vi "Setting GUI.vi"(3 "Path_In":path=path "C:/Users/mclmcgill/Desktop/Stroke_Perceptual_Testing") -> (0 "error out":errorcluster)   [LabVIEW 2012]
uses:
  Global_var.vi
  <userlib>/dhd_sdk7/dhd_sdk7.lvlib
panel:
  in  "Extreme Direction":u8=45 max=40 step=5
  in  "Get_center":bool
  out "Message":string
  out "after_str":string
  out "cur_path":path
  out "Center":dbl[](array[numeric]) format="%#_3g"
  in  "Alignment":bool
  in  "Quit":bool
  in  "Load":bool
  in  "Save":bool
  in  "Language":bool
  in  "Movement Distance":u8=15 max=40 step=5
  in  "Participant's Last Name":string
  in  "Participant's First Name":string
  # "cm"
  # "Recorded Center Position"
  # "degree"
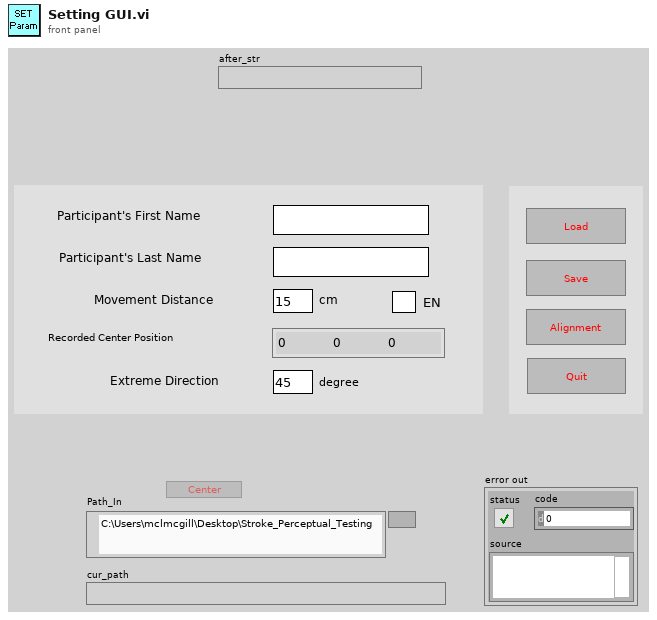
[diagram p1: front panel]
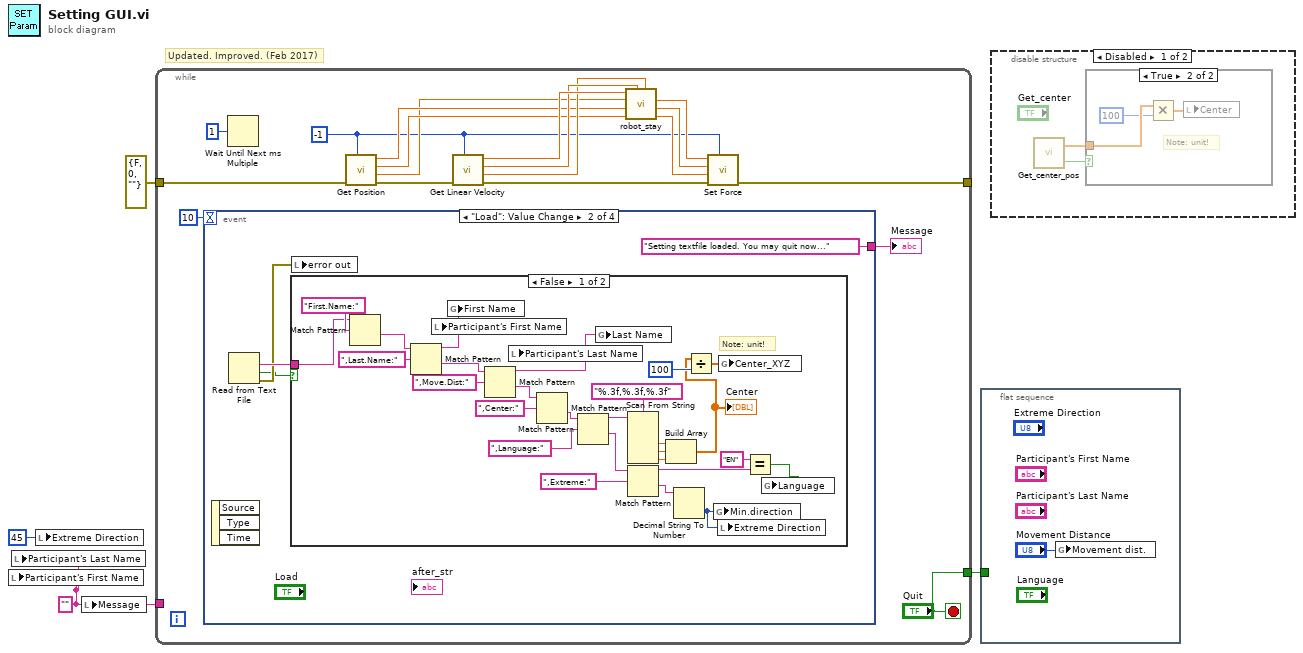
[diagram p0: block diagram]
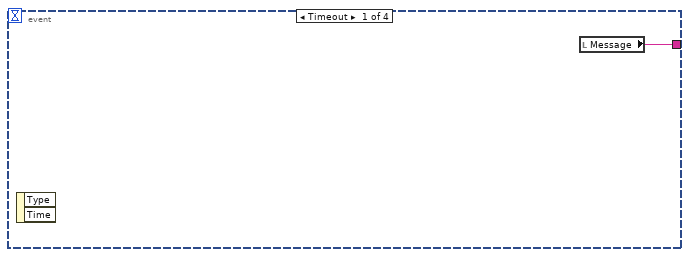
[diagram p4: hidden frame]
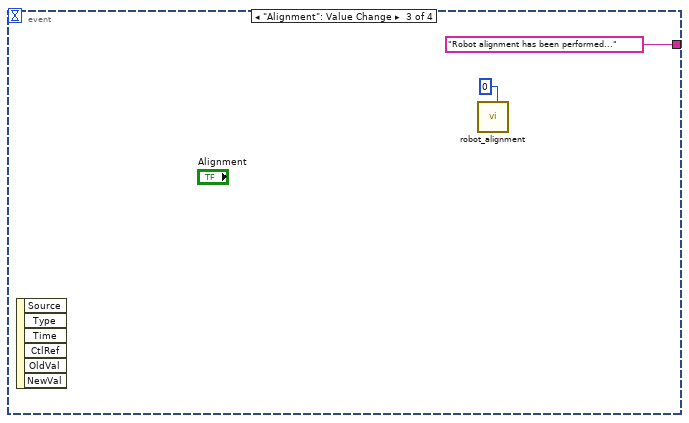
[diagram p6: hidden frame]
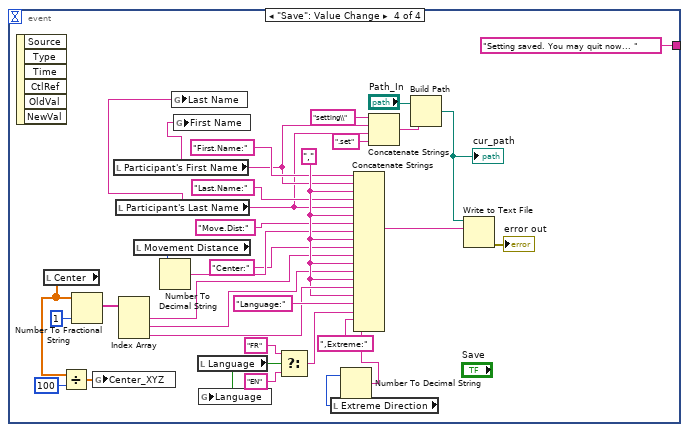
[diagram p7: hidden frame]
diagram:
  w2 = "" ("Message")
  # "Updated. Improved. (Feb 2017)"
  n1 = local write "Participant's First Name"(w2) -> ()
  n2 = local write "Participant's Last Name"(w2) -> ()
  n3 = local write "Extreme Direction"(u8 45 ("Extreme Direction")) -> ()
  n4 = local write "Message"(w2) -> ()
  n5 = while {
    tunnel: ["Quit"] -> w4
    tunnel: w2 -> [_]
    tunnel: errorcluster {"status"=FALSE, "code"=0, "source"=""} ("error") -> [w7]
    tunnel: [w5] -> _
    stop <- "Quit" stop-if-true
    w6 = i8 -1 ("millisecond multiple")
    n6 = event shown="[1] \"Load\": Value Change" {
      selector: _ -> [_ _ _ _]
      dyn-events: _ -> [_ _ _ _]
      timeout: 10 -> [_ _ _ _]
      tunnel: [w23 "Setting textfile loaded. You may quit now..." "Robot alignment has been performed..." "Setting saved. You may quit now... "] -> w19
      event Timeout {
        n7 = event-data() -> ()  [unwired: 1 in, 2 out]
        n8 = local read "Message"() -> (w23:string)
      }
      event "Load": Value Change {
        n9 = event-data() -> ()  [unwired: 1 in, 3 out]
        n10 = Read from Text File() -> (text=w27:string, cancelled=w24:bool, error out=w26:errorcluster)  [unwired: 4 in, 1 out]
        n11 = case shown="False" w24 {
          tunnel: w27 -> [w47 _]
          frame False {
            # "Note: unit!"
            n12 = Match Pattern(string=w47, regular expression="First.Name:") -> (after substring=w50:string)  [unwired: 1 in, 3 out]
            n13 = Match Pattern(string=w50, regular expression=",Last.Name:") -> (before substring=w37:string, after substring=w52:string)  [unwired: 1 in, 2 out]
            n14 = local write "Participant's First Name"(w37) -> ()
            n15 = global write "Global_var.vi" "First Name"(w37) -> ()
            n16 = Match Pattern(string=w52, regular expression=",Move.Dist:") -> (before substring=w36:string, after substring=w54:string)  [unwired: 1 in, 2 out]
            n17 = local write "Participant's Last Name"(w36) -> ()
            n18 = Match Pattern(string=w54, regular expression=",Center:") -> (after substring=w46:string)  [unwired: 1 in, 3 out]
            n19 = Match Pattern(string=w46, regular expression=",Language:") -> (before substring=w44:string, after substring=w39:string)  [unwired: 1 in, 2 out]
            n20 = global write "Global_var.vi" "Last Name"(w36) -> ()
            n21 = Scan From String(format string="%.3f,%.3f,%.3f", input string=w44) -> (output 1=w43:dbl, output 2=w42:dbl, output 3=w41:dbl)  [unwired: 5 in, 3 out]
            n22 = Match Pattern(string=w39, regular expression=",Extreme:") -> (before substring=w31:string, after substring=w32:string)  [unwired: 1 in, 2 out]
            n23 = Build Array(w43, w42, w41) -> (w33:dbl[])
            "Center" <- w33
            n24 = Decimal String To Number(string=w32) -> (number=w28:i32)  [unwired: 2 in, 1 out]
            n25 = Divide(x=w33, y=100) -> (x/y=w35:dbl[])
            n26 = global write "Global_var.vi" "Min.direction"(w28) -> ()
            n27 = local write "Extreme Direction"(w28) -> ()
            n28 = global write "Global_var.vi" "Center_XYZ"(w35) -> ()
            n29 = Equal?(x="EN", y=w31) -> (x = y?=w29:bool)
            n30 = global write "Global_var.vi" "Language"(w29) -> ()
          }
          frame True {
          }
        }
        n31 = local write "error out"(w26) -> ()
      }
      event "Alignment": Value Change {
        n32 = event-data() -> ()  [unwired: 1 in, 6 out]
        n33 = call "robot_alignment.vi"("Direction"=i8 0) -> ()  [unwired: 9 in]
      }
      event "Save": Value Change {
        w85 = ","
        n34 = event-data() -> ()  [unwired: 1 in, 6 out]
        n35 = local read "Center"() -> (w59:dbl[])
        n36 = Divide(x=w59, y=100) -> (x/y=w61:dbl[])
        n37 = Number To Fractional String(number=w59, precision (6)=i16 1 ("width (-)")) -> (F-format string=w82:string[])  [unwired: 2 in]
        n38 = global write "Global_var.vi" "Center_XYZ"(w61) -> ()
        n39 = local read "Participant's First Name"() -> (w63:string)
        n40 = local read "Participant's Last Name"() -> (w62:string)
        n41 = Index Array(array=w82) -> (element #1=w83:string, element #2=w84:string, element #3=w86:string)  [unwired: 3 in]
        n42 = local read "Movement Distance"() -> (w75:u8)
        n43 = Number To Decimal String(number=w75) -> (decimal integer string=w76:string)  [unwired: 1 in]
        n44 = global write "Global_var.vi" "Last Name"(w62) -> ()
        n45 = global write "Global_var.vi" "First Name"(w63) -> ()
        n46 = local read "Language"() -> (w58:bool)
        n47 = global write "Global_var.vi" "Language"(w58) -> ()
        n48 = Select(t="FR", s=w58, f="EN") -> (s? t:f=w88:string)
        n49 = local read "Extreme Direction"() -> (w57:u8)
        n50 = Number To Decimal String(number=w57) -> (decimal integer string=w64:string)  [unwired: 1 in]
        n51 = Concatenate Strings("First.Name:", w63, w85, "Last.Name:", w62, w85, "Move.Dist:", w76, w85, "Center:", w83, w85, w84, w85, w86, w85, "Language:", w88, ",Extreme:", w64) -> (w70:string)
        n52 = Concatenate Strings("setting\\" ("string"), w63, w62, ".set" ("string")) -> (w79:string)
        n53 = Build Path(base path="Path_In", name or relative path=w79) -> (appended path=w78:path)
        "cur_path" <- w78
        n54 = Write to Text File(file (use dialog)=w78, text=w70) -> (error out=→"error out":errorcluster)  [unwired: 2 in, 2 out]
      }
    }
    "Message" <- w19
    n55 = Wait Until Next ms Multiple(millisecond multiple=u32 1) -> ()  [unwired: 1 out]
    n56 = call <userlib>:"Get Position.vi"("ID"=w6, "error in (no error)"=w7) -> ("error out"=w18:errorcluster, "pz out"=w8:dbl, "py out"=w9:dbl, "px out"=w10:dbl)  [unwired: 5 in, 1 out]
    n57 = call <userlib>:"Get Linear Velocity.vi"("ID"=w6, "error in (no error)"=w18) -> ("error out"=w17:errorcluster, "vz out"=w11:dbl, "vy out"=w12:dbl, "vx out"=w13:dbl)  [unwired: 5 in, 1 out]
    n58 = call "robot_stay.vi"("Vz"=w11, "Z"=w8, "Vy"=w12, "Y"=w9, "X"=w10, "Vx"=w13) -> ("Fz"=w14:dbl, "Fy"=w15:dbl, "Fx"=w16:dbl)  [unwired: 3 in]
    n59 = call <userlib>:"Set Force.vi"("ID"=w6, "error in (no error)"=w17, "fz"=w14, "fy"=w15, "fx"=w16) -> ("error out"=w5:errorcluster)  [unwired: 5 in, 1 out]
  }
  n60 = flat-sequence {
    tunnel: w4 -> [_]
    frame #0 {
      n61 = global write "Global_var.vi" "Movement dist."("Movement Distance") -> ()
    }
  }
  n62 = disable-structure shown="Disabled" {
    frame Disabled {
      n63 = call "Get_center_pos.vi"() -> ("Position"=w91:dbl[], "flag"=w92:bool)  [unwired: 1 in]
      n64 = case shown="True" w92 {
        tunnel: w91 -> [_ w95]
        frame False {
        }
        frame True {
          # "Note: unit!"
          n65 = Multiply(x=w95, y=100) -> (x*y=w94:dbl[])
          n66 = local write "Center"(w94) -> ()
        }
      }
    }
    frame Enabled {
    }
  }
